vi "DSF.Engine.Plugin.Get Transfer Group by ID.vi"(8 "error in (no error)":errorcluster, 10 "transfer group id":i32, 11 "Plugin in":refnum<class "DSF.Engine.Plugin.lvclass">) -> (0 "error out":errorcluster, 2 "Transfer Group":refnum<class "DSF.Engine.Transfer Group.lvclass">, 3 "Plugin out":refnum<class "DSF.Engine.Plugin.lvclass">)   [LabVIEW 2017, in "DSF.Engine.lvlib" / "DSF.Engine.Plugin.lvclass"]
uses:
  DSF.Engine.Plugin.lvclass
  Transfer/DSF.Engine.Transfer Group.lvclass
  DSF.Engine.Plugin.lvclass/DSF.Engine.Plugin.ctl
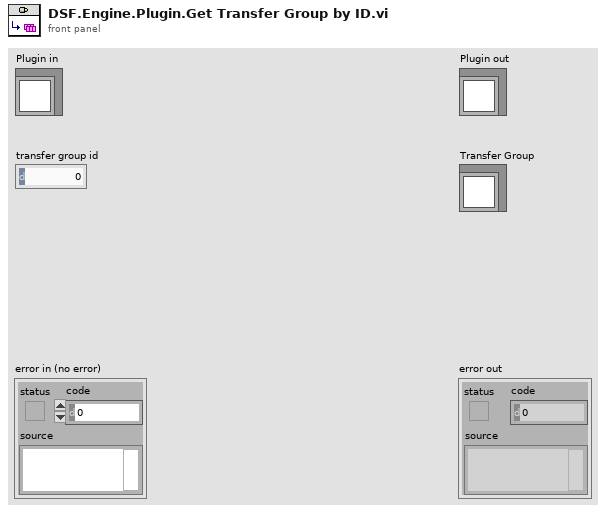
[diagram p1: front panel]
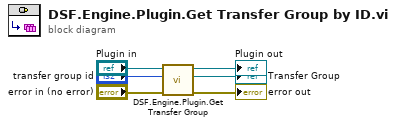
[diagram p0: block diagram]
diagram:
  n1 = call "DSF.Engine.Plugin.Get Transfer Group.vi"("transfer group id"="transfer group id", "Plugin in"="Plugin in") -> ("Transfer Group"=→"Transfer Group":refnum<class "DSF.Engine.Transfer Group.lvclass">, "Plugin out"=→"Plugin out":refnum<class "DSF.Engine.Plugin.lvclass">)  [unwired: 8 in]
  "error out" <- "error in (no error)"
